vi "RT_Angle_Of_Attack_in_DLR_Navigation_Reference_System_vcomp(SubVI)_2.vi"(8 "i":i32, 9 "V_wind [m/s]":dbl[][](array[numeric]), 10 "Rotation":T1, 11 "input cluster":T2) -> (0 "Speed_direction [rad]":dbl[](array[numeric]), 2 "AoA_yaw (rad)":dbl, 3 "AoA_pitch (rad)":dbl)   [LabVIEW 2017]
uses:
  <vilib>/Analysis/coordinate.llb/Euler Rotation Order.ctl
  <vilib>/Analysis/_algsub.llb/Vector Norm Type.ctl
  <vilib>/Analysis/_algsub.llb/Real Vector Norm.vi
  <vilib>/Analysis/NI_AALPro.lvlib
panel:
  out "Quaternion without roll":dbl[](array[numeric])
  out "Elevation [deg]":dbl
  out "Azimuth [deg]":dbl
  out "appended array":dbl[](array[numeric])
  out "Speed_quat":dbl[](array[numeric])
  out "Speed_pitch (rad)":dbl
  out "Speed_yaw (rad)":dbl
  out "v":dbl[](array[numeric])
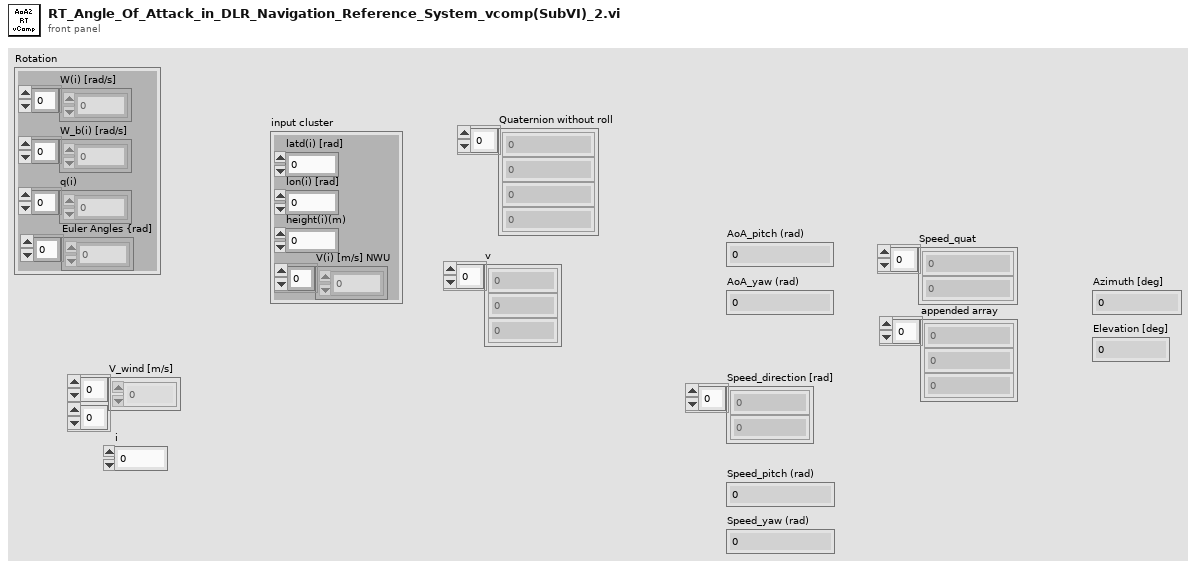
[diagram p1: front panel]
types:
  T1 = cluster{"W(i) [rad/s]":dbl[], "W_b(i) [rad/s]":dbl[], "q(i)":dbl[], "Euler Angles {rad]":dbl[]}
  T2 = cluster{"latd(i) [rad]":dbl, "lon(i) [rad]":dbl, "height(i)(m)":dbl, "V(i) [m/s] NWU":dbl[]}
  T3 = typedef "NI_AALPro.lvlib/Euler Rotation Order.ctl" = u16
  T4 = typedef "NI_AALPro.lvlib/Vector Norm Type.ctl" = u16
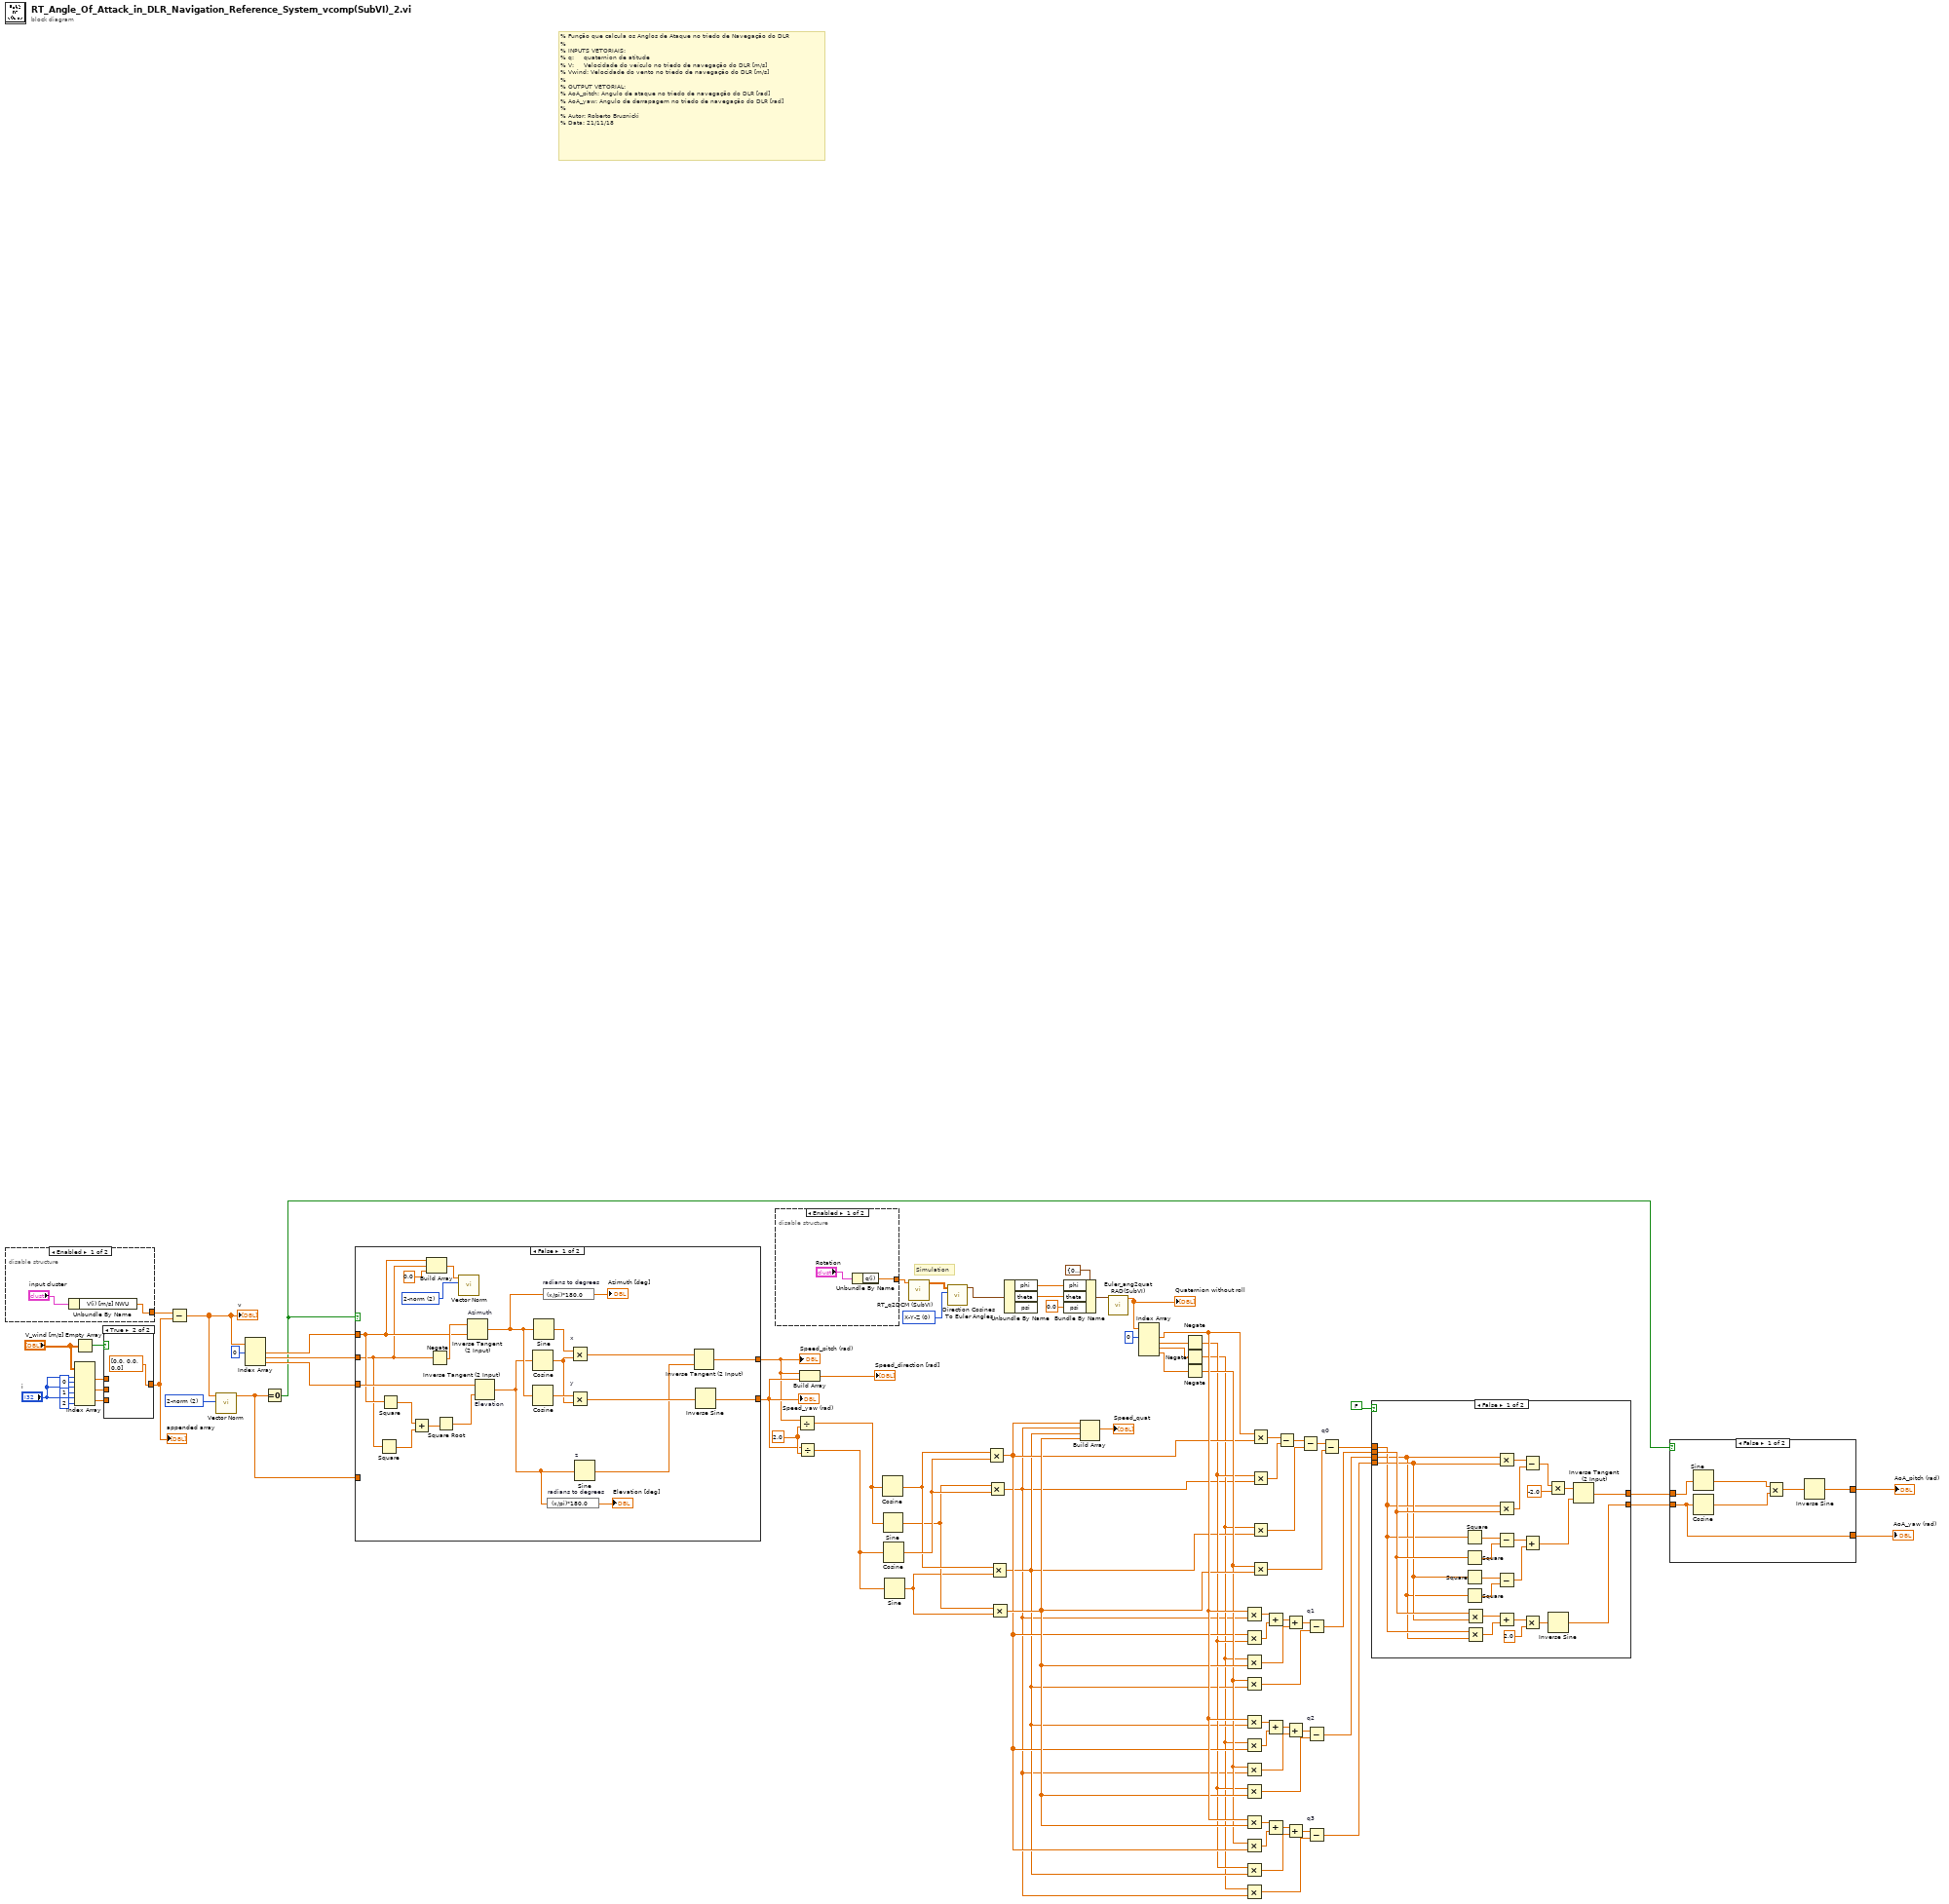
[diagram p0: block diagram]
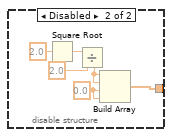
[diagram p2: hidden frame]
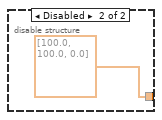
[diagram p3: hidden frame]
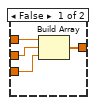
[diagram p4: hidden frame]
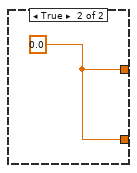
[diagram p5: hidden frame]
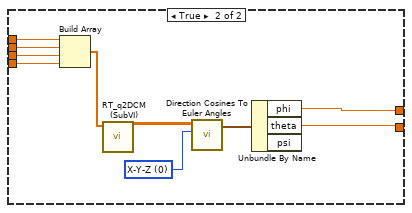
[diagram p6: hidden frame]
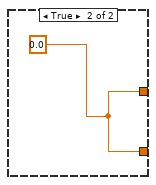
[diagram p7: hidden frame]
diagram:
  w12 = T3 0 items=["X-Y-Z", "X-Z-Y", "Y-X-Z", "Y-Z-X", "Z-X-Y", "Z-Y-X", "X-Y-X", "X-Z-X", "Y-X-Y", "Y-Z-Y", "Z-X-Z", "Z-Y-Z"] ("rotation order")
  w69 = 2.0 ("y")
  w75 = T4 2 items=["1-norm"=1, "2-norm"=2, "Inf-norm"=3, "-Inf-norm"=4, "User Defined"=5] ("norm type")
  # "Simulation"
  # "% Função que calcula os Anglos de Ataque no triedo de Navegação do DLR \n%\n% INPUTS VETORIAIS: \n% q:     quaternion de atitude   \n% V:     Velocidade do veículo no triedo de navegação do DLR [m/s]\n% Vwind: Velocidade do vento no triedo de navegação do DLR [m/s]\n%\n% OUTPUT VETORIAL:\n% AoA_pitch: Angulo de ataque no triedo de navegação do DLR [rad]\n% AoA_yaw: Angulo de derrapagem no triedo de navegação do DLR [rad]\n%\n% Autor: Roberto Brusnicki\n% Data: 21/11/18"
  n1 = disable-structure shown="Enabled" {
    disable-tunnel: [w87 dbl[] [100.0, 100.0, 0.0] ("V (m/s)")] -> w84
    frame Enabled {
      n2 = Unbundle By Name("input cluster") -> ("V(i) [m/s] NWU"=w87:dbl[])
    }
    frame Disabled {
    }
  }
  n3 = Index Array(array="V_wind [m/s]", index (row) #1="i", index (col) #1=0 ("disabled index (col)"), index (row) #2="i", index (col) #2=1 ("disabled index (col)"), index (row) #3="i", index (col) #3=2 ("disabled index (col)")) -> (element #1=w79:dbl, element #2=w78:dbl, element #3=w77:dbl)
  n4 = Empty Array?(array="V_wind [m/s]") -> (empty?=w8:bool)
  n5 = case shown="True" w8 {
    tunnel: w79 -> [w92 _]
    tunnel: w78 -> [w91 _]
    tunnel: w77 -> [w90 _]
    tunnel: [w89 dbl[] [0.0, 0.0, 0.0]] -> w76
    frame False {
      n6 = Build Array(w92, w91, w90) -> (w89:dbl[])
    }
    frame True {
    }
  }
  "appended array" <- w76
  n7 = Subtract(x=w84, y=w76) -> (x-y=w74:dbl[])
  "v" <- w74
  n8 = call-poly <vilib>:"Vector Norm.vi"("norm type"=w75, "Input Vector"=w74) -> ("norm"=w71:dbl)  [unwired: 8 in, 1 out]
  n9 = Index Array(array=w74, index #1=0 ("index (row)")) -> (element #1=w73:dbl, element #2=w72:dbl, element #3=w18:dbl)  [unwired: 2 in]
  n10 = Equal To 0?(x=w71) -> (x = 0?=w16:bool)
  n11 = case shown="False" w16 {
    tunnel: [w107 w117] -> w68
    tunnel: [w104 w117] -> w67
    tunnel: w73 -> [w97 _]
    tunnel: w72 -> [w96 _]
    tunnel: w71 -> [_ _]
    tunnel: w18 -> [w115 _]
    frame False {
      w114 = T4 2 items=["1-norm"=1, "2-norm"=2, "Inf-norm"=3, "-Inf-norm"=4, "User Defined"=5] ("norm type")
      n12 = Square(x=w96) -> (x^2=w99:dbl)
      n13 = Square(x=w97) -> (x^2=w98:dbl)
      n14 = Add(x=w98, y=w99) -> (x+y=w95:dbl)
      n15 = Build Array(w97, w96, 0.0 ("element")) -> (w112:dbl[])
      n16 = Negate(x=w96) -> (-x=w116:dbl)
      n17 = Square Root(x=w95) -> (sqrt(x)=w94:dbl)
      n18 = call-poly <vilib>:"Vector Norm.vi"("norm type"=w114, "Input Vector"=w112) -> ()  [unwired: 8 in, 2 out]
      n19 = Inverse Tangent (2 Input) "Azimuth"(1:w97, 2:w116) -> (0:w103:dbl)
      n20 = Inverse Tangent (2 Input) "Elevation"(1:w94, 2:w115) -> (0:w100:dbl)
      n21 = Cosine(x=w100) -> (cos(x)=w109:dbl)
      n22 = Cosine(x=w103) -> (cos(x)=w110:dbl)
      n23 = Sine(x=w103) -> (sin(x)=w111:dbl)
      n24 = expression code="(x/pi)*180.0" "radians to degrees"(w103) -> (→"Azimuth [deg]":dbl)
      n25 = expression code="(x/pi)*180.0" "radians to degrees"(w100) -> (→"Elevation [deg]":dbl)
      n26 = Multiply "x"(x=w111, y=w109) -> (x*y=w106:dbl)
      n27 = Multiply "y"(x=w110, y=w109) -> (x*y=w108:dbl)
      n28 = Sine "z"(x=w100) -> (sin(x)=w105:dbl)
      n29 = Inverse Tangent (2 Input)(1:w105, 2:w106) -> (0:w104:dbl)
      n30 = Inverse Sine(1:w108) -> (0:w107:dbl)
    }
    frame True {
      w117 = 0.0 ("Speed_pitch (rad)")
    }
  }
  "Speed_pitch (rad)" <- w67
  "Speed_yaw (rad)" <- w68
  n31 = disable-structure shown="Enabled" {
    disable-tunnel: [w119 w125] -> w10
    frame Enabled {
      n32 = Unbundle By Name("Rotation") -> ("q(i)"=w119:dbl[])
    }
    frame Disabled {
      w120 = 0.0 ("element")
      n33 = Square Root(x=2.0) -> (sqrt(x)=w123:dbl)
      n34 = Divide(x=w123, y=2.0) -> (x/y=w121:dbl)
      n35 = Build Array(w121, w121, w120, w120) -> (w125:dbl[])
    }
  }
  n36 = Divide(x=w67, y=w69) -> (x/y=w66:dbl)
  n37 = Divide(x=w68, y=w69) -> (x/y=w65:dbl)
  n38 = Build Array(w67, w68) -> (→"Speed_direction [rad]":dbl[])
  n39 = Cosine(x=w66) -> (cos(x)=w63:dbl)
  n40 = Sine(x=w66) -> (sin(x)=w62:dbl)
  n41 = Cosine(x=w65) -> (cos(x)=w64:dbl)
  n42 = Sine(x=w65) -> (sin(x)=w61:dbl)
  n43 = call "RT_q2DCM (SubVI).vi"("Quaternion"=w10) -> ("DCM"=w11:dbl[][])  [unwired: 10 in]
  n44 = call <vilib>:"Direction Cosines To Euler Angles.vi"("rotation order"=w12, "Direction Cosines"=w11) -> ("Euler Angles"=w1:cluster{"phi":dbl, "theta":dbl, "psi":dbl})  [unwired: 8 in, 1 out]
  n45 = Multiply(x=w63, y=w64) -> (x*y=w29:dbl)
  n46 = Multiply(x=w62, y=w64) -> (x*y=w25:dbl)
  n47 = Multiply(x=w63, y=w61) -> (x*y=w27:dbl)
  n48 = Multiply(x=w62, y=w61) -> (x*y=w31:dbl)
  n49 = Unbundle By Name(w1) -> ("phi"=w5:dbl, "theta"=w6:dbl)  [unwired: 1 out]
  n50 = Bundle By Name(cluster=cluster{"phi":dbl, "theta":dbl, "psi":dbl} {"phi"=0.0, "theta"=0.0, "psi"=0.0} ("Euler Angles 2"), "phi"=w5, "theta"=w6, "psi"=0.0) -> (w3:cluster{"phi":dbl, "theta":dbl, "psi":dbl})
  n51 = Build Array(w29, w25, w27, w31) -> (→"Speed_quat":dbl[])
  n52 = call "Euler_ang2quat RAD(SubVI).vi"("Euler Angles [rad]"=w3) -> ("Quaternions"=w2:dbl[])  [unwired: 10 in]
  "Quaternion without roll" <- w2
  n53 = Index Array(array=w2, index #1=0 ("index")) -> (element #1=w32:dbl, element #2=w57:dbl, element #3=w58:dbl, element #4=w59:dbl)  [unwired: 3 in]
  n54 = Negate(x=w57) -> (-x=w28:dbl)
  n55 = Negate(x=w58) -> (-x=w26:dbl)
  n56 = Negate(x=w59) -> (-x=w30:dbl)
  n57 = Multiply(x=w32, y=w25) -> (x*y=w50:dbl)
  n58 = Multiply(x=w29, y=w28) -> (x*y=w49:dbl)
  n59 = Multiply(x=w26, y=w31) -> (x*y=w46:dbl)
  n60 = Multiply(x=w30, y=w27) -> (x*y=w45:dbl)
  n61 = Multiply(x=w32, y=w27) -> (x*y=w39:dbl)
  n62 = Multiply(x=w26, y=w29) -> (x*y=w40:dbl)
  n63 = Multiply(x=w30, y=w25) -> (x*y=w43:dbl)
  n64 = Multiply(x=w28, y=w31) -> (x*y=w44:dbl)
  n65 = Multiply(x=w32, y=w31) -> (x*y=w38:dbl)
  n66 = Multiply(x=w30, y=w29) -> (x*y=w37:dbl)
  n67 = Multiply(x=w28, y=w27) -> (x*y=w34:dbl)
  n68 = Multiply(x=w26, y=w25) -> (x*y=w33:dbl)
  n69 = Multiply(x=w32, y=w29) -> (x*y=w56:dbl)
  n70 = Multiply(x=w28, y=w25) -> (x*y=w55:dbl)
  n71 = Multiply(x=w26, y=w27) -> (x*y=w53:dbl)
  n72 = Multiply(x=w30, y=w31) -> (x*y=w51:dbl)
  n73 = Add(x=w50, y=w49) -> (x+y=w48:dbl)
  n74 = Add(x=w39, y=w40) -> (x+y=w41:dbl)
  n75 = Add(x=w38, y=w37) -> (x+y=w36:dbl)
  n76 = Subtract(x=w56, y=w55) -> (x-y=w54:dbl)
  n77 = Add(x=w48, y=w46) -> (x+y=w47:dbl)
  n78 = Add(x=w41, y=w43) -> (x+y=w42:dbl)
  n79 = Add(x=w36, y=w34) -> (x+y=w35:dbl)
  n80 = Subtract(x=w54, y=w53) -> (x-y=w52:dbl)
  n81 = Subtract "q1"(x=w47, y=w45) -> (x-y=w23:dbl)
  n82 = Subtract "q2"(x=w42, y=w44) -> (x-y=w22:dbl)
  n83 = Subtract "q3"(x=w35, y=w33) -> (x-y=w21:dbl)
  n84 = Subtract "q0"(x=w52, y=w51) -> (x-y=w24:dbl)
  n85 = case shown="False" FALSE {
    tunnel: w24 -> [w133 w158]
    tunnel: w23 -> [w135 w157]
    tunnel: w22 -> [w132 w156]
    tunnel: w21 -> [w134 w155]
    tunnel: [w136 w153] -> w20
    tunnel: [w126 w152] -> w19
    frame False {
      n86 = Square(x=w133) -> (x^2=w143:dbl)
      n87 = Square(x=w135) -> (x^2=w142:dbl)
      n88 = Square(x=w134) -> (x^2=w141:dbl)
      n89 = Square(x=w132) -> (x^2=w140:dbl)
      n90 = Multiply(x=w135, y=w134) -> (x*y=w131:dbl)
      n91 = Multiply(x=w133, y=w132) -> (x*y=w130:dbl)
      n92 = Multiply(x=w132, y=w134) -> (x*y=w148:dbl)
      n93 = Multiply(x=w133, y=w135) -> (x*y=w147:dbl)
      n94 = Subtract(x=w143, y=w142) -> (x-y=w139:dbl)
      n95 = Subtract(x=w141, y=w140) -> (x-y=w138:dbl)
      n96 = Add(x=w131, y=w130) -> (x+y=w128:dbl)
      n97 = Subtract(x=w148, y=w147) -> (x-y=w146:dbl)
      n98 = Add(x=w139, y=w138) -> (x+y=w137:dbl)
      n99 = Multiply(x=w128, y=2.0) -> (x*y=w127:dbl)
      n100 = Multiply(x=w146, y=-2.0) -> (x*y=w144:dbl)
      n101 = Inverse Sine(1:w127) -> (0:w126:dbl)
      n102 = Inverse Tangent (2 Input)(1:w137, 2:w144) -> (0:w136:dbl)
    }
    frame True {
      w150 = T3 0 items=["X-Y-Z", "X-Z-Y", "Y-X-Z", "Y-Z-X", "Z-X-Y", "Z-Y-X", "X-Y-X", "X-Z-X", "Y-X-Y", "Y-Z-Y", "Z-X-Z", "Z-Y-Z"] ("rotation order")
      n103 = Build Array(w158, w157, w156, w155) -> (w154:dbl[])
      n104 = call "RT_q2DCM (SubVI).vi"("Quaternion"=w154) -> ("DCM"=w151:dbl[][])  [unwired: 10 in]
      n105 = call <vilib>:"Direction Cosines To Euler Angles.vi"("rotation order"=w150, "Direction Cosines"=w151) -> ("Euler Angles"=w149:cluster{"phi":dbl, "theta":dbl, "psi":dbl})  [unwired: 8 in, 1 out]
      n106 = Unbundle By Name(w149) -> ("phi"=w153:dbl, "theta"=w152:dbl)  [unwired: 1 out]
    }
  }
  n107 = case shown="False" w16 {
    tunnel: w20 -> [w164 _]
    tunnel: [w160 w165] -> w15
    tunnel: w19 -> [w159 _]
    tunnel: [w159 w165] -> w14
    frame False {
      n108 = Sine(x=w164) -> (sin(x)=w163:dbl)
      n109 = Cosine(x=w159) -> (cos(x)=w162:dbl)
      n110 = Multiply(x=w163, y=w162) -> (x*y=w161:dbl)
      n111 = Inverse Sine(1:w161) -> (0:w160:dbl)
    }
    frame True {
      w165 = 0.0
    }
  }
  "AoA_pitch (rad)" <- w15
  "AoA_yaw (rad)" <- w14
